vi "Config-Sweep-Const-Source.vi"(6 "compliance (SMUs only)":dbl=0.0001 format="%^.2e", 8 "error in (no error)":errorcluster, 9 "source (V or A)":dbl format="%^.3e", 10 "unit (SMU1:0)":u16(ring) items=["SMU 1", "SMU2", "SMU3", "SMU4", "SMU5", "SMU6", "VSU1", "VSU2"], 11 "VISA session":refnum<visa-resource-name>) -> (0 "error out":errorcluster, 3 "VISA resource name out":refnum<visa-resource-name>)   [LabVIEW 2016, in "Agilent 415X Series.lvlib"]
doc: "This VI configures one constant source unit which can be an SMU or a VSU. The selected unit (channel) must be configured as a CONSTANT source and its mode may not be COMMON, otherwise the instrument will return an error.\n\n* This VI only checks for the existence of SMU5/6 should one of \nthem be selected as the unit to be configured. This VI does NOT check whether the selected unit is in CONSTANT mode."
uses:
  Agilent 415X Series.lvlib
panel:
  # "This VI should only be used to set up a\nchannel in CONSTANT(but not COMMON) mode"
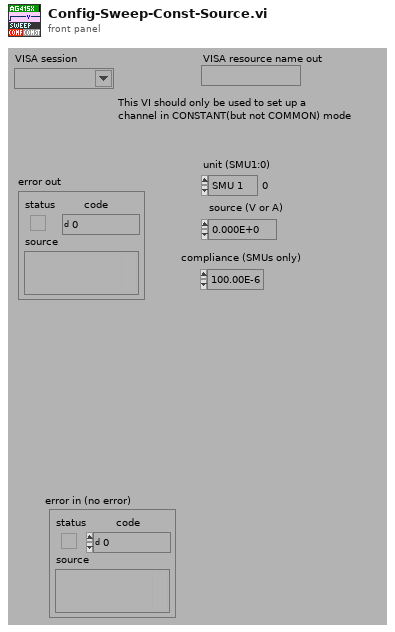
[diagram p1: front panel]
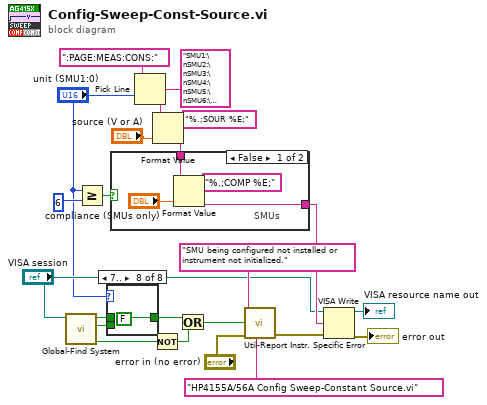
[diagram p0: block diagram]
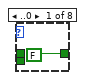
[diagram p2: hidden frame]
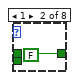
[diagram p3: hidden frame]
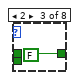
[diagram p4: hidden frame]
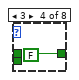
[diagram p5: hidden frame]
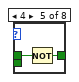
[diagram p6: hidden frame]
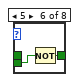
[diagram p7: hidden frame]
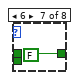
[diagram p8: hidden frame]
diagram:
  n1 = call "Global-Find System.vi"("VISA session"="VISA session") -> ("found"=w8:bool, "SMU6 present"=w13:bool, "SMU5 present"=w11:bool)  [unwired: 3 in, 5 out]
  n2 = Greater Or Equal?(x="unit (SMU1:0)", y=6) -> (x >= y?=w16:bool)
  n3 = case shown="7.." "unit (SMU1:0)" {
    tunnel: [FALSE FALSE FALSE FALSE w29 w31 FALSE FALSE] -> w10
    tunnel: w13 -> [_ _ _ _ _ w30 _ _]
    tunnel: w11 -> [_ _ _ _ w28 _ _ _]
    frame ..0 {
    }
    frame 1 {
    }
    frame 2 {
    }
    frame 3 {
    }
    frame 4 {
      n4 = Not(x=w28) -> (.not. x?=w29:bool)
    }
    frame 5 {
      n5 = Not(x=w30) -> (.not. x?=w31:bool)
    }
    frame 6 {
    }
    frame 7.. {
    }
  }
  n6 = Pick Line(string ("")=":PAGE:MEAS:CONS:", multi-line string="SMU1:\nSMU2:\nSMU3:\nSMU4:\nSMU5:\nSMU6:\nVSU1:\nVSU2:", line index="unit (SMU1:0)") -> (output string=w20:string)
  n7 = Not(x=w8) -> (.not. x?=w7:bool)
  n8 = Format Value(string ("")=w20, format string="%.;SOUR %E;", value (0)="source (V or A)") -> (output string=w17:string)
  n9 = case shown="False" w16 {
    tunnel: w17 -> [w35 w38]
    tunnel: [w34 w38] -> w14
    frame False {
      # "SMUs"
      n10 = Format Value(string ("")=w35, format string="%.;COMP %E;", value (0)="compliance (SMUs only)") -> (output string=w34:string)
    }
    frame True {
      # "VSUs"
    }
  }
  n11 = Or(x=w10, y=w7) -> (x .or. y?=w9:bool)
  n12 = call "Util-Report Instr. Specific Error.vi"("source"="HP4155A/56A Config Sweep-Constant Source.vi", "error in (no error)"="error in (no error)", "error message"="SMU being configured not installed or instrument not initialized.", "new error"=w9) -> ("error out"=w3:errorcluster)  [unwired: 6 in, 1 out]
  n13 = VISA Write(VISA resource name="VISA session", write buffer=w14, error in (no error)=w3) -> (VISA resource name out=→"VISA resource name out":refnum<visa-resource-name>, error out=→"error out":errorcluster)  [unwired: 1 out]
